vi "error.Write code.vi"(8 "error in (no error)":errorcluster, 10 "code":i32, 11 "error in":refnum<class "error.lvclass">) -> (0 "error out":errorcluster, 3 "error out":refnum<class "error.lvclass">)   [LabVIEW 2016, in "error.lvclass"]
uses:
  error.lvclass
  error.lvclass/error.ctl
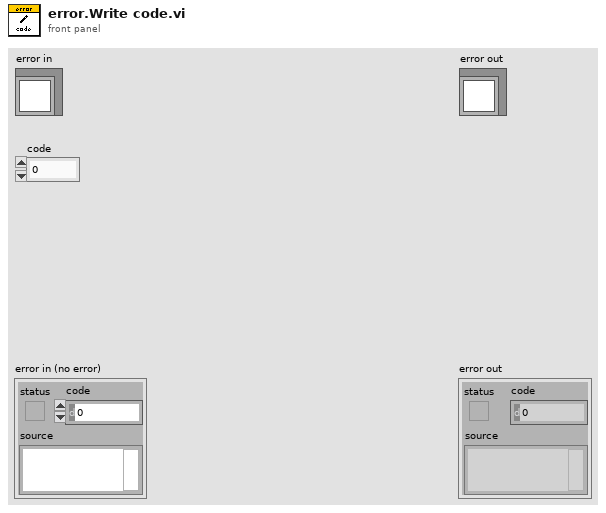
[diagram p1: front panel]
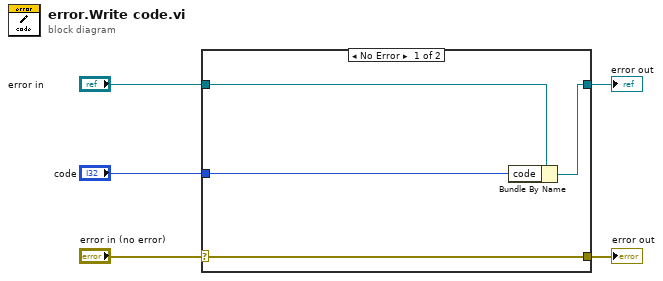
[diagram p0: block diagram]
diagram:
  n1 = case shown="No Error" "error in (no error)" {
    selector: "error in (no error)" -> [w9 w10]
    tunnel: [w9 w10] -> w4
    tunnel: [w7 w11] -> w2
    tunnel: "error in" -> [w8 w11]
    tunnel: "code" -> [w6 _]
    frame No Error {
      n2 = Bundle By Name(cluster=w8, "code"=w6) -> (w7:refnum<class "error.lvclass">)
    }
    frame Error {
    }
  }
  "error out" <- w4
  "error out" <- w2
